vi "Write Bearer.vi"(8 "error in (no error)":errorcluster, 10 "Bearer":string, 11 "Guardian in":refnum<class "Guardian.lvclass">) -> (0 "error out":errorcluster, 3 "Guardian out":refnum<class "Guardian.lvclass">)   [LabVIEW 2026, in "TALOS.lvlib" / "Guardian.lvlib" / "Guardian.lvclass"]
uses:
  Guardian.lvclass
  Guardian.lvclass/Guardian.ctl
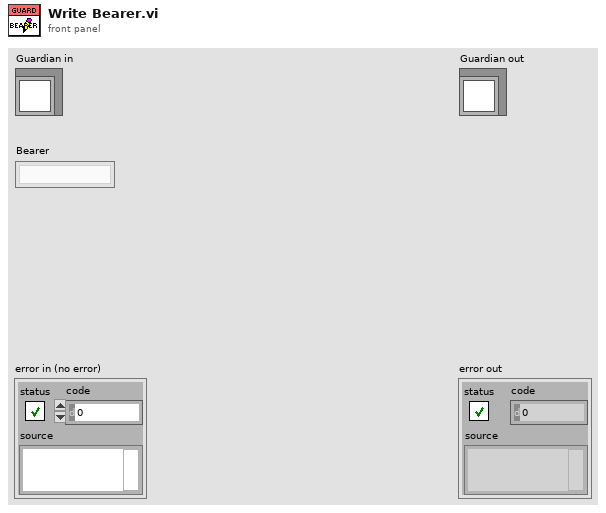
[diagram p1: front panel]
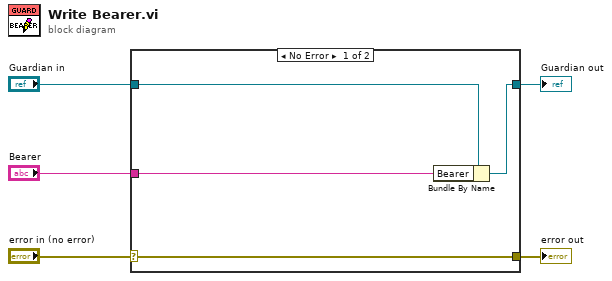
[diagram p0: block diagram]
diagram:
  n1 = case shown="No Error" "error in (no error)" {
    selector: "error in (no error)" -> [w9 w10]
    tunnel: [w9 w10] -> w4
    tunnel: [w7 w11] -> w2
    tunnel: "Guardian in" -> [w8 w11]
    tunnel: "Bearer" -> [w6 _]
    frame No Error {
      n2 = Bundle By Name(cluster=w8, "Bearer"=w6) -> (w7:refnum<class "Guardian.lvclass">)
    }
    frame Error {
    }
  }
  "error out" <- w4
  "Guardian out" <- w2
